vi "VSI Write Read Bytes.vi"(5 "ReadLen":u16, 6 "WriteLen":u16, 7 "pWriteData":u8[](array[numeric])=array[10240 elements], 9 "SPIIndex":i32, 10 "DevIndex":i32, 11 "DevType":i32) -> (2 "function return":i32, 3 "pReadData":u8[](array[numeric]))   [LabVIEW 2010, in "ControlSPI.lvlib"]
doc: "int WINAPI VSI_WriteReadBytes(int DevType,int DevIndex,int SPIIndex,unsigned char* pWriteData,unsigned short WriteLen,unsigned char * pReadData,unsigned short ReadLen);"
uses:
  ControlSPI.lvlib
  ControlSPI/Ginkgo_Driver.dll
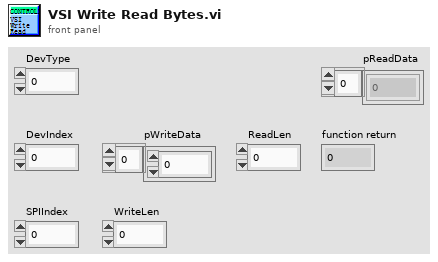
[diagram p1: front panel]
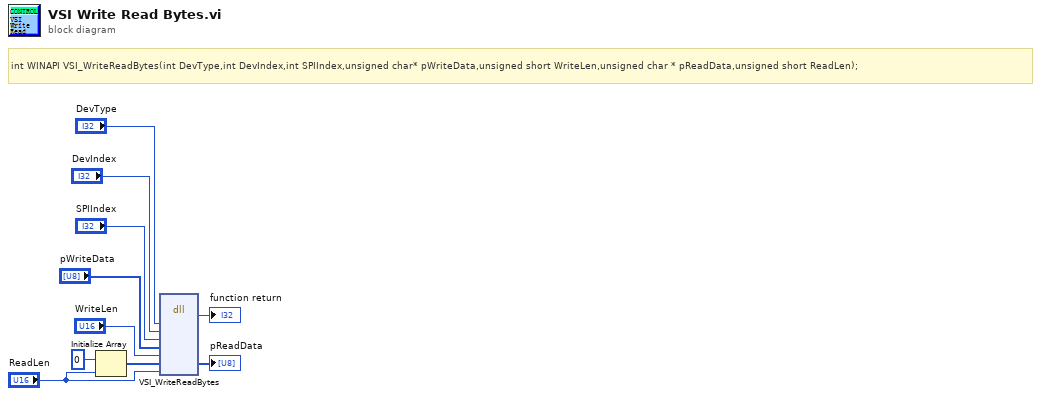
[diagram p0: block diagram]
diagram:
  # "int WINAPI VSI_WriteReadBytes(int DevType,int DevIndex,int SPIIndex,unsigned char* pWriteData,unsigned short WriteLen,unsigned char * pReadData,unsigned short ReadLen);"
  n1 = Initialize Array(u8 0 ("element"), "ReadLen") -> (w4:u8[])
  n2 = dll-call lib="E:/Project/vt_ginkgo/truck/Ginkgo Driver/vs2010/Ginkgo_USB-I2C&SPI&CAN_API_v2.0.3.3/lib/labview_32bit/ControlSPI/Ginkgo_Driver.*" fn="VSI_WriteReadBytes"("DevType"="DevType", "DevIndex"="DevIndex", "SPIIndex"="SPIIndex", "pWriteData"="pWriteData", "WriteLen"="WriteLen", "pReadData"=w4, "ReadLen"="ReadLen") -> (→"function return":i32, "pReadData"=→"pReadData":u8[])  [unwired: 9 in, 2 out]
